vi "strobe_digital_in_to_file.vi"(11 "Path":path) -> ()   [LabVIEW 2016]
panel:
  out "Stim ID":dbl
  out "StimTrigger":bool
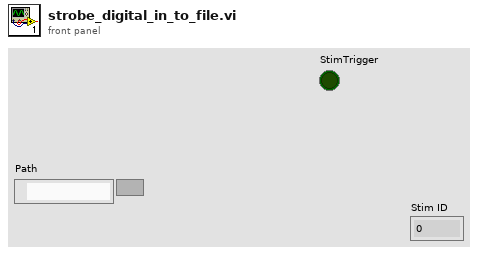
[diagram p1: front panel]
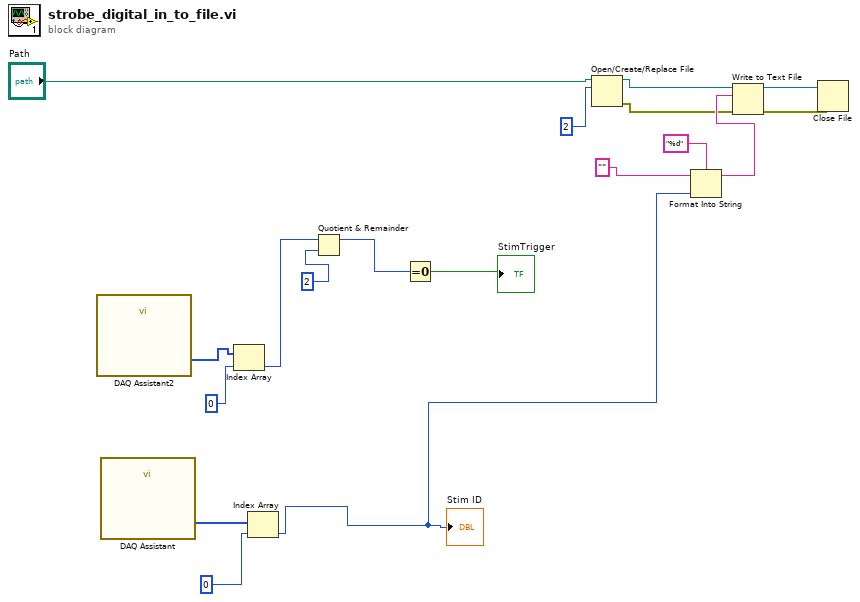
[diagram p0: block diagram]
diagram:
  n1 = call "DAQ Assistant2"() -> ("data"=w16:u32[])  [unwired: 17 in, 2 out]
  n2 = call "DAQ Assistant"() -> ("data"=w17:u32[])  [unwired: 17 in, 2 out]
  n3 = Index Array(array=w16, index=0) -> (element=w14:u32)
  n4 = Index Array(array=w17, index=0) -> (element=w6:u32)
  "Stim ID" <- w6
  n5 = Quotient & Remainder(x=w14, y=2) -> (x-y*floor(x/y)=w12:u32)  [unwired: 1 out]
  n6 = Equal To 0?(x=w12) -> (x = 0?=→"StimTrigger":bool)
  n7 = Open/Create/Replace File(file path (use dialog)="Path", operation (0:open)=2) -> (refnum out=w10:refnum<file>, error out=w3:errorcluster)  [unwired: 4 in, 1 out]
  n8 = Format Into String(format string="%d", initial string="", w6) -> (resulting string=w5:string)  [unwired: 1 in, 1 out]
  n9 = Write to Text File(file (use dialog)=w10, text=w5, error in=w3) -> (refnum out=w2:refnum<file>, error out=w4:errorcluster)  [unwired: 1 in, 1 out]
  n10 = Close File(refnum=w2, error in=w4) -> ()  [unwired: 2 out]
